vi "verify parameters generic.vi"(8 "error in (no error)":errorcluster, 11 "Simulated_CCD_Camera in":refnum<class "Sim_Ixon_Ultra.lvclass">) -> (0 "error out":errorcluster, 3 "Simulated_CCD_Camera out":refnum<class "Sim_Ixon_Ultra.lvclass">)   [LabVIEW 2018, in "Sim_Ixon_Ultra.lvclass"]
uses:
  Sim_Ixon_Ultra.lvclass
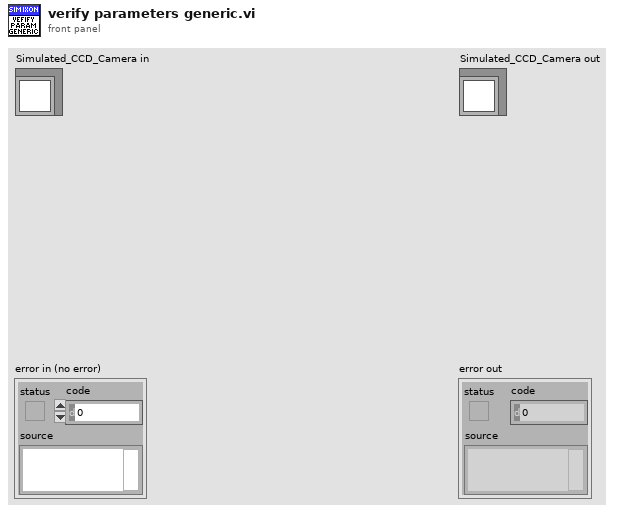
[diagram p1: front panel]
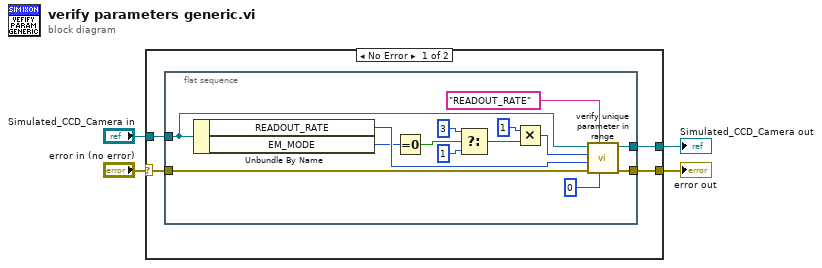
[diagram p0: block diagram]
diagram:
  n1 = case shown="No Error" "error in (no error)" {
    selector: "error in (no error)" -> [w8 w24]
    tunnel: [w5 w24] -> w3
    tunnel: [w6 w23] -> w1
    tunnel: "Simulated_CCD_Camera in" -> [w7 w23]
    frame No Error {
      n2 = flat-sequence {
        tunnel: w8 -> [w22]
        tunnel: w7 -> [w21]
        tunnel: [w10] -> w6
        tunnel: [w9] -> w5
        frame #0 {
          n3 = Unbundle By Name(w21) -> ("READOUT_RATE"=w19:u16, "EM_MODE"=w14:u16)
          n4 = Equal To 0?(x=w14) -> (x = 0?=w15:bool)
          n5 = Select(t=3, s=w15, f=1) -> (s? t:f=w16:i32)
          n6 = Multiply(x=1, y=w16) -> (x*y=w11:i32)
          n7 = call "verify unique parameter in range.vi"("lower limit"=0, "parameter name"="READOUT_RATE", "error in (no error)"=w22, "value"=w19, "upper limit"=w11, "Simulated_CCD_Camera in"=w21) -> ("error out"=w9:errorcluster, "Simulated_CCD_Camera out"=w10:refnum<class "Sim_Ixon_Ultra.lvclass">)  [unwired: 4 in]
        }
      }
    }
    frame Error {
    }
  }
  "error out" <- w3
  "Simulated_CCD_Camera out" <- w1
